vi "Get DAQ Dev Info Stub.vi"(1 "Numeric":u32, 2 "Numeric 2":u32) -> (0 "information string":string)   [LabVIEW 2020]
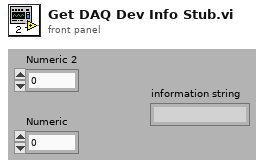
[diagram p1: front panel]
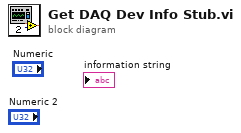
[diagram p0: block diagram]
diagram:
